vi "2.1.vi"() -> ()   [LabVIEW 2013]
panel:
  out "Array":dbl[](array[numeric])
  out "Numeric 2":dbl
  in  "Numeric":dbl
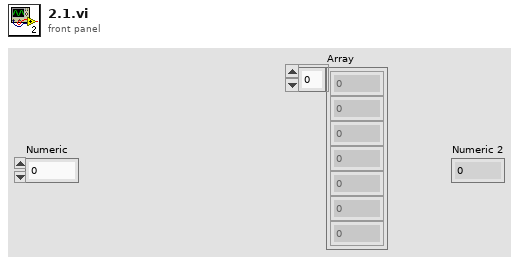
[diagram p1: front panel]
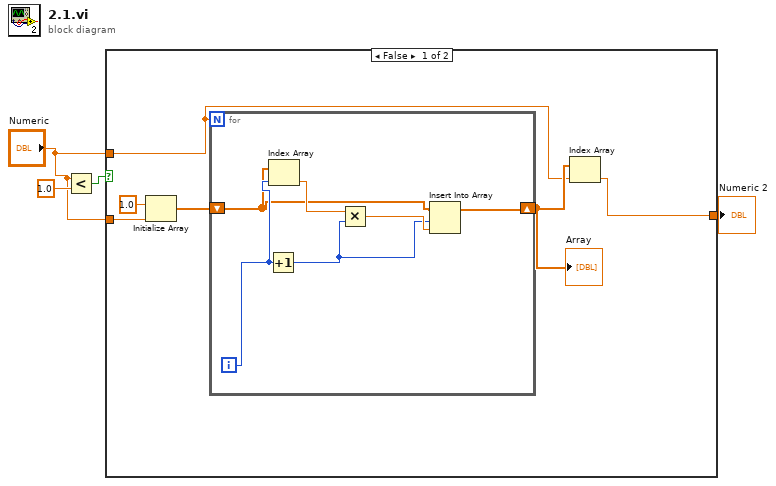
[diagram p0: block diagram]
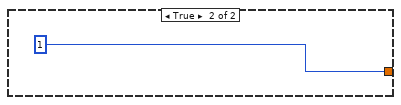
[diagram p2: hidden frame]
diagram:
  n1 = Less?(x="Numeric", y=1.0) -> (x < y?=w3:bool)
  n2 = case shown="False" w3 {
    tunnel: "Numeric" -> [w5 _]
    tunnel: "Numeric" -> [w7 _]
    tunnel: [w6 1] -> w1
    frame False {
      n3 = Initialize Array(1.0 ("element"), w5) -> (w9:dbl[])
      n4 = for {
        N: w7 -> [_]
        shift-right: [w14] -> w8
        shift-left: w9 -> [w11]
        i -> [w13]
        n5 = Increment(x=w13) -> (x+1=w15:i32)
        n6 = Index Array(array=w11, index=w13) -> (element=w12:dbl)
        n7 = Multiply(x=w12, y=w15) -> (x*y=w16:dbl)
        n8 = Insert Into Array(array=w11, index=w15, new element=w16) -> (w14:dbl[])
      }
      "Array" <- w8
      n9 = Index Array(array=w8, index=w7) -> (element=w6:dbl)
    }
    frame True {
    }
  }
  "Numeric 2" <- w1
